vi "Get SMO HELP getAll.vi"(8 "error in (no error)":errorcluster, 11 "instrument.PPMS in":refnum<class "instrument.PPMS.lvclass">) -> (0 "error out":errorcluster, 2 "response cluster":variant, 3 "instrument.PPMS out":refnum<class "instrument.PPMS.lvclass">)   [LabVIEW 2019, in "instrument.PPMS.lvclass"]
uses:
  instrument.PPMS.lvclass
  Typedefs/PPMS.getAll--cluster.ctl
  <vilib>/PRIrvin/JSON-Schema/JSON-Schema.lvlib
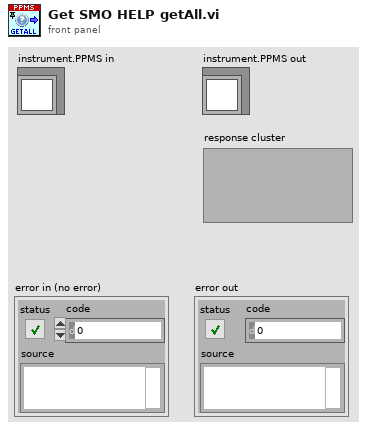
[diagram p1: front panel]
types:
  T1 = typedef "instrument.PPMS.lvclass/PPMS.getAll--cluster.ctl" = cluster{"Chamber Status":string, "Helium Level":dbl, "Temperature":dbl, "Temperature Status":string, "Magnetic Field":dbl, "Magnet Status":string, "Position":dbl}
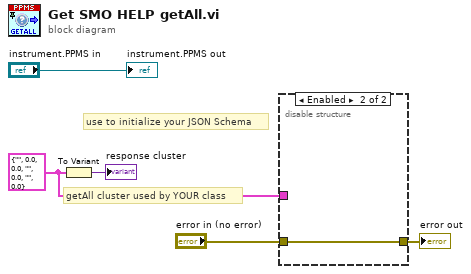
[diagram p0: block diagram]
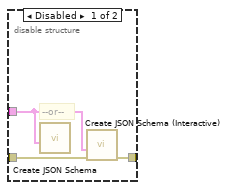
[diagram p2: hidden frame]
diagram:
  w1 = T1 {"Chamber Status"="", "Helium Level"=0.0, "Temperature"=0.0, "Temperature Status"="", "Magnetic Field"=0.0, "Magnet Status"="", "Position"=0.0} ("getAll")
  # "use to initialize your JSON Schema"
  # "getAll cluster used by YOUR class"
  n1 = To Variant(anything=w1) -> (Variant=→"response cluster":variant)
  n2 = disable-structure shown="Enabled" {
    disable-tunnel: w1 -> [w6 _]
    disable-tunnel: "error in (no error)" -> [w8 w9]
    disable-tunnel: [w7 w9] -> w5
    frame Disabled {
      # "--or--"
      n3 = call <vilib>:"Create JSON Schema.vi"("LV Object"=w6) -> ()  [unwired: 10 in, 1 out]
      n4 = call <vilib>:"Create JSON Schema (Interactive).vi"("error in (no error)"=w8, "LV Object"=w6) -> ("error out"=w7:errorcluster)  [unwired: 8 in, 1 out]
    }
    frame Enabled {
    }
  }
  "error out" <- w5
  "instrument.PPMS out" <- "instrument.PPMS in"
